vi "Inspect Errors.vi"(8 "error in (no error)":errorcluster, 11 "Fault Monitor in":refnum<class "Fault Monitor.lvclass">) -> (0 "error out":errorcluster, 3 "Fault Monitor out":refnum<class "Fault Monitor.lvclass">)   [LabVIEW 2023, in "Fault Monitor.lvlib" / "Fault Monitor.lvclass"]
uses:
  Library/Fault Monitor.lvclass
  Library/Fault Monitor.lvclass/Fault Monitor.ctl
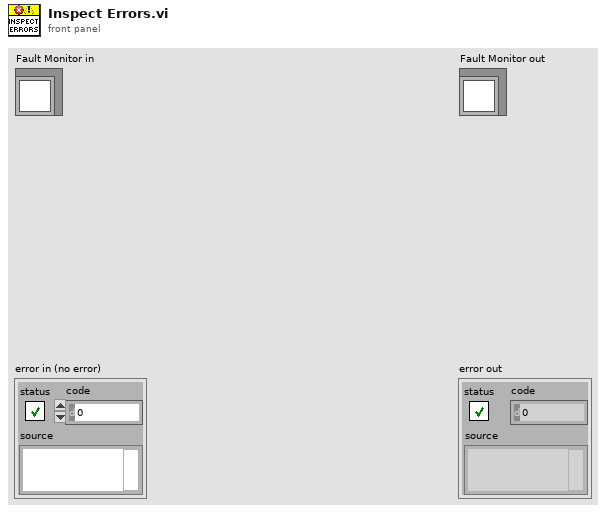
[diagram p1: front panel]
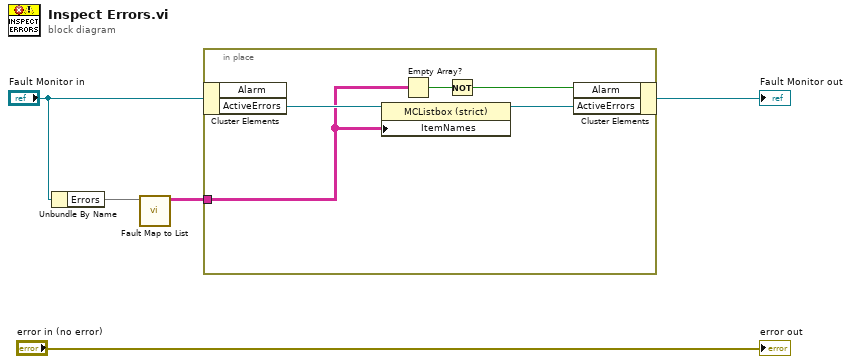
[diagram p0: block diagram]
diagram:
  n1 = Unbundle By Name("Fault Monitor in") -> ("Errors"=w4:map{string, errorcluster[]})
  n2 = call "Fault Map to List.vi"("Fault map in"=w4) -> ("List out"=w1:string[][])  [unwired: 10 in]
  n3 = in-place {
    in-place-border: w1 -> [w7]
    n4 = in-place-cluster #1("Fault Monitor in") -> ("ActiveErrors"=w10:refnum<vi>)  [unwired: 1 out]
    n5 = property class="MCListbox (strict)"(reference=w10, "ItemNames"=w7) -> (reference out=w9:refnum<vi>)  [unwired: 1 in, 1 out]
    n6 = Empty Array?(array=w7) -> (empty?=w8:bool)
    n7 = Not(x=w8) -> (.not. x?=w6:bool)
    n8 = in-place-cluster #1("Alarm"=w6, "ActiveErrors"=w9) -> (→"Fault Monitor out":refnum<class "Fault Monitor.lvclass">)
  }
  "error out" <- "error in (no error)"
